vi "Test Comm.vi"() -> ()   [LabVIEW 2012]
uses:
  <vilib>/FPGAPlugInAG/cRIO-9081/niLvFpga_Open_cRIO-9081.vi
  <vilib>/rvi/interface/common/dynamic/niFpgaDynamicAddResources.vi
  <vilib>/Utility/error.llb/Error Cluster From Error Code.vi
  <vilib>/rvi/errors/niLvFpgaAdjustHostInterfaceError.vi
  <vilib>/FPGAPlugInAG/Dynamic/niLvFpga_Close_Dynamic.vi
  <vilib>/rvi/interface/nirviOpenFPGA/nirviOpenFPGA.xnode
  FPGA Bitfiles/Nicholas_FPGATarget_FPGAExe_9Amsex+uXF0.lvbitx
  <vilib>/rvi/interface/nirviMethod/nirviMethod.xnode
  <vilib>/rvi/interface/nirviReadWriteControl/nirviReadWriteControl.xnode
  <vilib>/rvi/interface/nirviCloseFPGA/nirviCloseFPGA.xnode
  <vilib>/rvi/interface/Simulation/niFpgaSimulationCallBeginRW.vi
  NiFpgaLv.dll
  <vilib>/FPGAPlugInAG/Dynamic/niLvFpga_ConfigureFifo_Dynamic.vi
  <vilib>/rvi/errors/niLvFpgaMergeErrorWithErrorCode.vi
  <vilib>/FPGAPlugInAG/Dynamic/niLvFpga_StartFifo_Dynamic.vi
  <vilib>/FPGAPlugInAG/Dynamic/niLvFpga_ReadFifo_Dynamic.vi
panel:
  out "Waveform Chart":u32(graph)
  out "x-y 2":u32
  out "Elements Remaining":u32
  out "Actual Depth":u32
  out "latch time":u32
  out "error out":errorcluster
  out "x-y":u32
  in  "Boolean":bool
  out "Waveform Graph":dbl[](graph)
  out "Loop Rate Out":u32
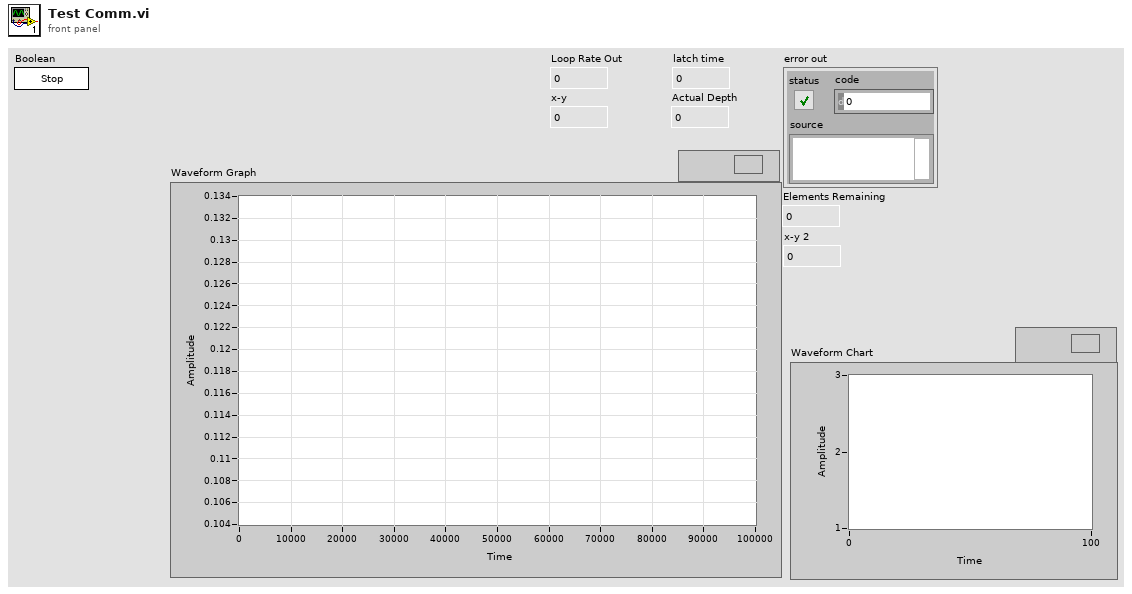
[diagram p1: front panel]
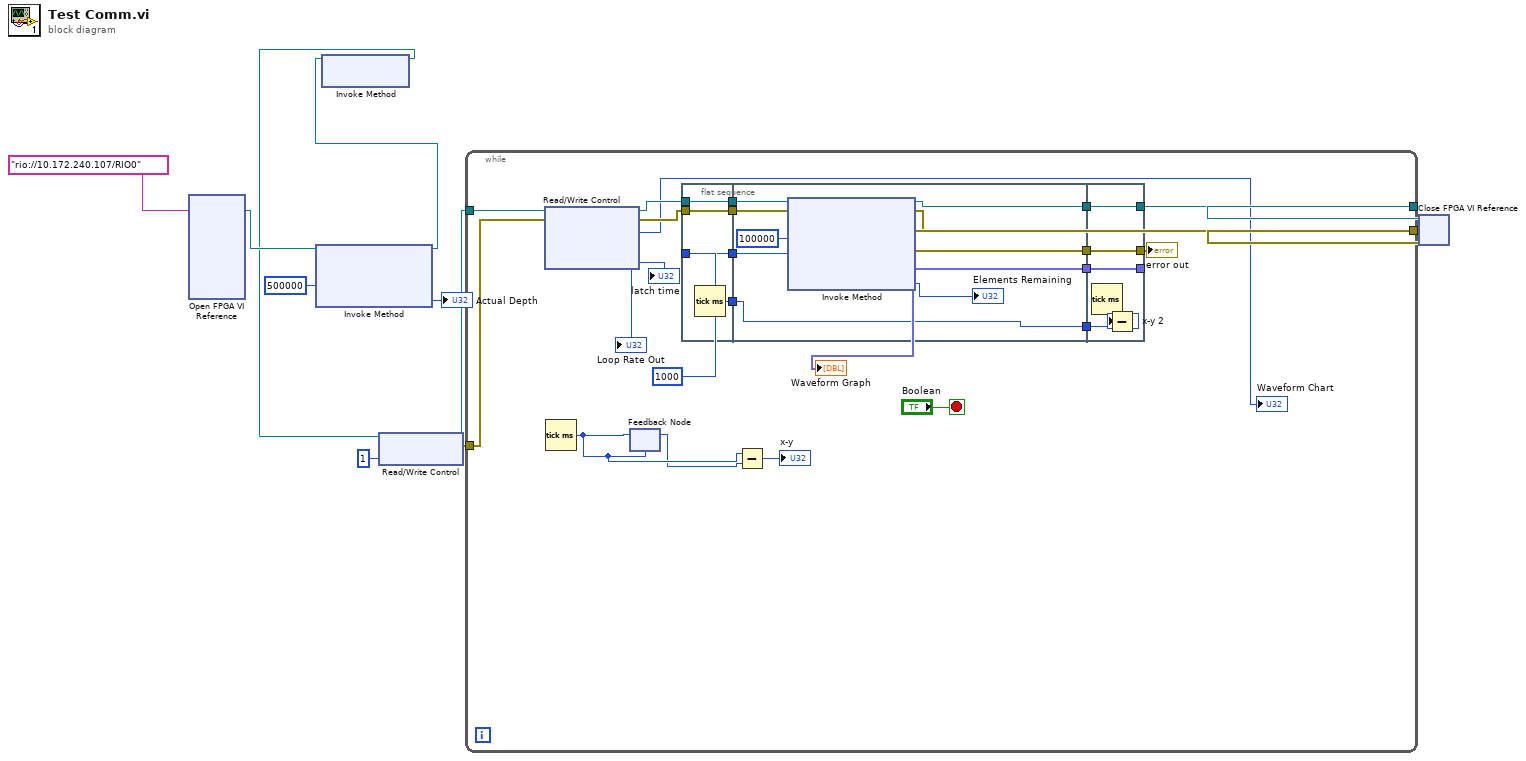
[diagram p0: block diagram]
diagram:
  n1 = xnode "Open FPGA VI Reference"("resource name"=tag "rio://10.172.240.107/RIO0") -> ("FPGA VI Reference Out"=w5:refnum<k20>)  [unwired: 1 in, 1 out]
  n2 = xnode "Invoke Method"("FPGA VI Reference In"=w5, "Requested Depth"=u32 500000) -> ("FPGA VI Reference Out"=w2:refnum<k20>, "Actual Depth"=→"Actual Depth":u32)  [unwired: 1 in, 1 out]
  n3 = xnode "Invoke Method"("FPGA VI Reference In"=w2) -> ("FPGA VI Reference Out"=w1:refnum<k20>)  [unwired: 1 in, 1 out]
  n4 = xnode "Read/Write Control"("FPGA VI Reference In"=w1, "Loop Rate In"=u32 1) -> ("FPGA VI Reference Out"=w10:refnum<k20>, "error out"=w6:errorcluster)  [unwired: 1 in]
  n5 = while {
    tunnel: w10 -> [w33]
    tunnel: [w22] -> w8
    tunnel: [w21] -> w7
    tunnel: w6 -> [w28]
    stop <- "Boolean" stop-if-true
    n6 = xnode "Read/Write Control"("FPGA VI Reference In"=w33, "error in"=w28) -> ("FPGA VI Reference Out"=w26:refnum<k20>, "error out"=w25:errorcluster, "Loop Rate Out"=→"Loop Rate Out" →"Waveform Chart":u32, "latch time"=→"latch time":u32)  [unwired: 1 out]
    n7 = Tick Count (ms)() -> (millisecond timer value=w31:u32)
    n8 = feedback-in #1(w31) -> ()
    n9 = feedback #1(w31) -> (w30:u32)
    n10 = flat-sequence {
      tunnel: 1000 ("Timeout (ms)") -> [w35]
      tunnel: w25 -> [w36]
      tunnel: w26 -> [w37]
      tunnel: [w37] -> w17
      tunnel: [w36] -> w16
      tunnel: [w35] -> w15
      tunnel: [w34] -> w14
      tunnel: [w41] -> w20
      tunnel: [w40] -> w19
      tunnel: [w39] -> w18
      tunnel: w17 -> [w46]
      tunnel: w16 -> [w45]
      tunnel: w15 -> [w43]
      tunnel: w14 -> [w38]
      tunnel: [w38] -> w13
      tunnel: [w50] -> w21
      tunnel: [w51] -> w22
      tunnel: [w52] -> w23
      tunnel: w20 -> [w52]
      tunnel: w19 -> [w51]
      tunnel: w18 -> [w50]
      tunnel: w13 -> [w48]
      frame #0 {
        n11 = Tick Count (ms)() -> (millisecond timer value=w34:u32)
      }
      frame #1 {
        n12 = xnode "Invoke Method"("FPGA VI Reference In"=w46, "error in"=w45, "Number of Elements"=u32 100000, "Timeout (ms)"=w43) -> ("FPGA VI Reference Out"=w40:refnum<k20>, "error out"=w39:errorcluster, "Data"=w41:fxp<+/-,24,5>[], "Elements Remaining"=→"Elements Remaining":u32)
      }
      frame #2 {
        n13 = Tick Count (ms)() -> (millisecond timer value=w49:u32)
        n14 = Subtract(x=w49, y=w48) -> (x-y=→"x-y 2":u32)
      }
    }
    n15 = Subtract(x=w31, y=w30) -> (x-y=→"x-y":u32)
    "Waveform Graph" <- w23
    "error out" <- w21
  }
  n16 = xnode "Close FPGA VI Reference"("FPGA VI Reference In"=w8, "error in"=w7) -> ()  [unwired: 1 out]
